vi "ソース コード.vi"() -> ()   [LabVIEW 2014]
panel:
  in  "y":dbl=2.0 format="%#_13g"
  out "x+y":dbl
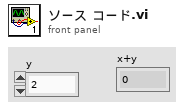
[diagram p1: front panel]
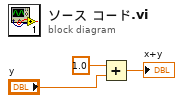
[diagram p0: block diagram]
diagram:
  n1 = Add(x=1.0, y="y") -> (x+y=→"x+y":dbl)
